vi "toStringArray.vi"(8 "error in (no error)":errorcluster, 11 "RampToneDown in":refnum<class "RampToneDown.lvclass">) -> (0 "error out":errorcluster, 2 "eventStringArray":string[](array[string]), 3 "RampToneDown out":refnum<class "RampToneDown.lvclass">)   [LabVIEW 2009, in "Tools.lvlib" / "Scripting.lvlib" / "RampToneDown.lvclass"]
uses:
  RampToneDown.lvclass
  RampTone/RampTone.lvclass
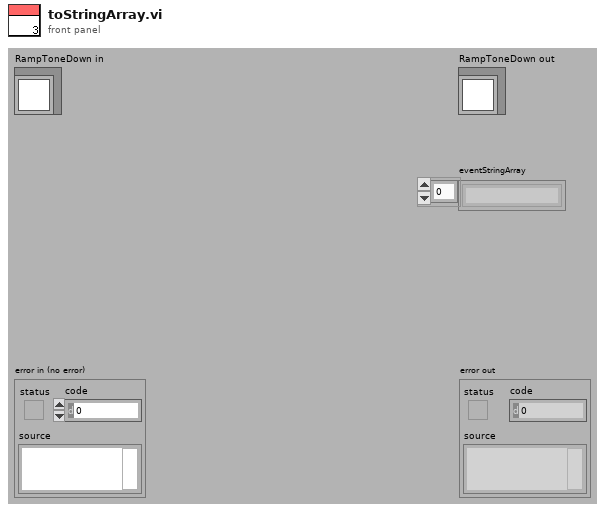
[diagram p1: front panel]
types:
  T1 = cluster{"rampTime":dbl, "timeStep":dbl, "dataValueStep":dbl}
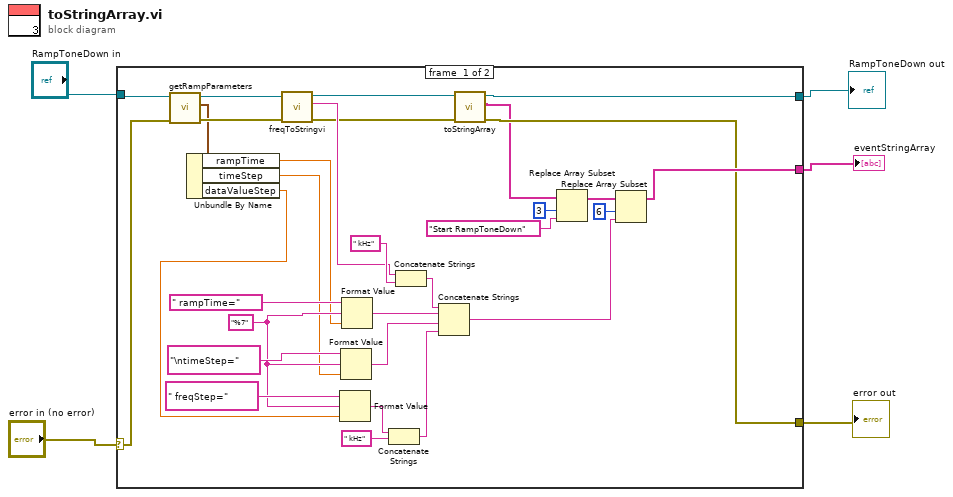
[diagram p0: block diagram]
diagram:
  n1 = case shown="No Error" "error in (no error)" {
    selector: "error in (no error)" -> [w16 w37]
    tunnel: [w7 w37] -> w1
    tunnel: [w23 _] -> w3
    tunnel: "RampToneDown in" -> [w15 w38]
    tunnel: [w9 w38] -> w2
    frame #0 {
      w22 = "%7"
      n2 = call "getRampParameters.vi"("error in (no error)"=w16, "RampTone in"=w15) -> ("error out"=w17:errorcluster, "RampParameters"=w14:T1, "RampTone out"=w18:refnum<class "RampToneDown.lvclass">)  [unwired: 7 in]
      n3 = Unbundle By Name(w14) -> ("rampTime"=w13:dbl, "timeStep"=w12:dbl, "dataValueStep"=w11:dbl)
      n4 = call-dynamic "freqToStringvi.vi"("error in (no error)"=w17, "SingleTone in"=w18) -> ("error out"=w8:errorcluster, "frequency"=w19:string, "SingleTone out"=w10:refnum<class "RampToneDown.lvclass">)  [unwired: 7 in]
      n5 = Format Value(string ("")=" freqStep=", format string=w22, value (0)=w11) -> (output string=w26:string)
      n6 = Format Value(string ("")="\ntimeStep=", format string=w22, value (0)=w12) -> (output string=w28:string)
      n7 = Format Value(string ("")=" rampTime=", format string=w22, value (0)=w13) -> (output string=w29:string)
      n8 = Concatenate Strings(w26, " kHz") -> (w24:string)
      n9 = Concatenate Strings(w19, " kHz") -> (w20:string)
      n10 = Concatenate Strings(w20, w29, w28, w24) -> (w27:string)
      n11 = call-parent "toStringArray.vi"("error in (no error)"=w8, "RampTone in"=w10) -> ("error out"=w7:errorcluster, "eventStringArray"=w6:string[], "RampTone out"=w9:refnum<class "RampToneDown.lvclass">)  [unwired: 7 in]
      n12 = Replace Array Subset(array=w6, new element="Start RampToneDown", index=3) -> (w32:string[])
      n13 = Replace Array Subset(array=w32, new element=w27, index=6) -> (w23:string[])
    }
    frame #1 {
    }
  }
  "error out" <- w1
  "RampToneDown out" <- w2
  "eventStringArray" <- w3
